vi "Level Hi Lo (SubVI).vi"(8 "Chan 0 trigger level lo (V)":dbl, 9 "Chan 0 trigger level hi (V)":dbl, 10 "trigger source (No longer used when we can trigger on any channel.)":u8, 11 "scaling coefficients":T3[](array[typedef])) -> (2 "configuration":T1={"level"=0.0, "trigger when"=enum."Trigger Below"}, 3 "configuration 2":T1)   [LabVIEW 2021, in "Device Session.lvclass"]
uses:
  Device Session.lvclass
  <instrlib>/_niInstr/Data Trigger/v1/Shared/Public/Level Configuration FXP(+-,18,1).ctl
  <instrlib>/_niInstr/Data Trigger/v1/Shared/Public/Level Configuration Trigger When.ctl
  <instrlib>/_niInstr/Multirecord Acquisition/Interface/v1/Host/Public/Scaling Coefficient.ctl
  <instrlib>/_niInstr/Data Trigger/v1/Shared/niInstr Data Trigger v1 Shared.lvlib
  <instrlib>/_niInstr/Multirecord Acquisition/Interface/v1/Host/niInstr Multirecord Acquisition v1 Host.lvclass
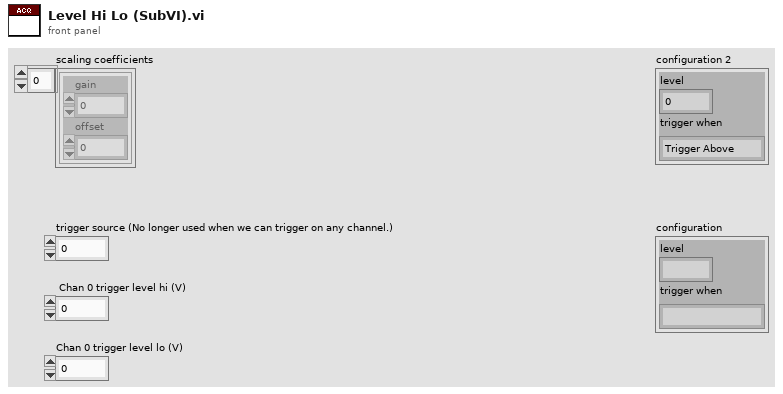
[diagram p1: front panel]
types:
  T1 = typedef "niInstr Data Trigger v1 Shared.lvlib/Level Configuration FXP(+-,18,1).ctl" = cluster{"level":fxp<+/-,18,5>, "trigger when":T2}
  T2 = typedef "niInstr Data Trigger v1 Shared.lvlib/Level Configuration Trigger When.ctl" = enum8{"Trigger Above", "Trigger Below"}
  T3 = typedef "niInstr Multirecord Acquisition v1 Host.lvclass/Scaling Coefficient.ctl" = cluster{"gain":dbl, "offset":dbl}
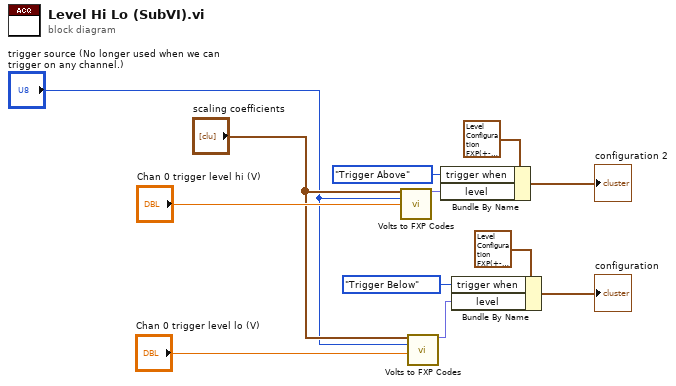
[diagram p0: block diagram]
diagram:
  n1 = call "Volts to FXP Codes.vi"("scaling coefficients"="scaling coefficients", "channel index"="trigger source (No longer used when we can trigger on any channel.)", "level (V)"="Chan 0 trigger level hi (V)") -> ("codes"=w3:fxp<+/-,18,1>)  [unwired: 12 in]
  n2 = call "Volts to FXP Codes.vi"("scaling coefficients"="scaling coefficients", "channel index"="trigger source (No longer used when we can trigger on any channel.)", "level (V)"="Chan 0 trigger level lo (V)") -> ("codes"=w6:fxp<+/-,18,1>)  [unwired: 12 in]
  n3 = Bundle By Name(cluster=T1 {"level"=0.0, "trigger when"=enum."Trigger Above"} ("configuration"), "trigger when"=Level_Configuration_Trigger_When."Trigger Above", "level"=w3) -> (→"configuration 2":T1)
  n4 = Bundle By Name(cluster=T1 {"level"=0.0, "trigger when"=enum."Trigger Above"} ("configuration"), "trigger when"=Level_Configuration_Trigger_When."Trigger Below", "level"=w6) -> (→"configuration":T1)
